vi "Format data da formato sql.vi"(11 "aaaa-mm-gg":string) -> (3 "String":string)   [LabVIEW 2019]
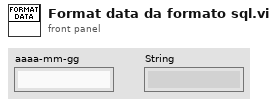
[diagram p1: front panel]
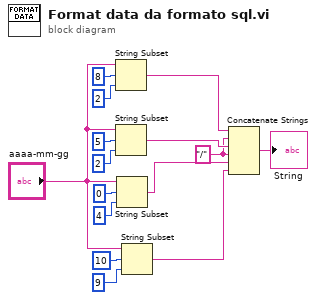
[diagram p0: block diagram]
diagram:
  w9 = "/" ("string")
  n1 = String Subset(string="aaaa-mm-gg", offset (0)=8, length (rest)=2 ("length (rest)")) -> (substring=w14:string)
  n2 = String Subset(string="aaaa-mm-gg", offset (0)=5, length (rest)=2 ("length (rest)")) -> (substring=w15:string)
  n3 = String Subset(string="aaaa-mm-gg", offset (0)=0, length (rest)=4 ("length (rest)")) -> (substring=w13:string)
  n4 = String Subset(string="aaaa-mm-gg", offset (0)=10, length (rest)=9 ("length (rest)")) -> (substring=w12:string)
  n5 = Concatenate Strings(w14, w9, w15, w9, w13, w12) -> (→"String":string)
